vi "UIGlobalVariable.vi"(4 "Enum":enum16{"Get", "Set"}(ring), 11 "Input":T1={"Play"=FALSE, "number of samples/ch"=100000, "sound format"={"sample rate (S/s)"=22050.0, "number of channels"=2, "bits per sample"=16}}) -> (3 "Output":T1={"Play"=FALSE, "number of samples/ch"=100000, "sound format"={"sample rate (S/s)"=22050.0, "number of channels"=2, "bits per sample"=16}})   [LabVIEW 2017]
uses:
  UIData.ctl
  <vilib>/sound2/lvsound2.llb/Sound Data Format.ctl
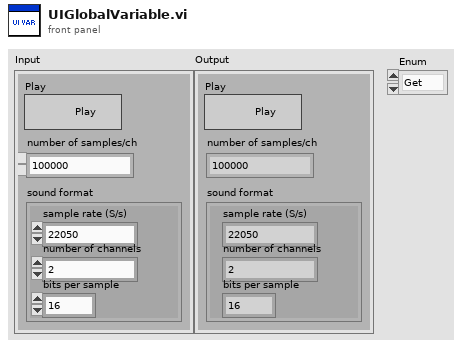
[diagram p1: front panel]
types:
  T1 = typedef "UIData.ctl" = cluster{"Play":bool, "number of samples/ch":i32, "sound format":T2}
  T2 = typedef "Sound Data Format.ctl" = cluster{"sample rate (S/s)":dbl, "number of channels":i32, "bits per sample":i32}
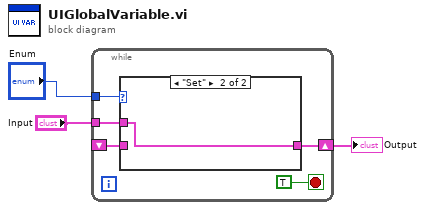
[diagram p0: block diagram]
diagram:
  n1 = while {
    tunnel: "Enum" -> [w8]
    tunnel: "Input" -> [w7]
    shift-right: [w5] -> w2
    shift-left: _ -> [w4]
    stop <- TRUE stop-if-true
    n2 = case shown="\"Set\"" w8 {
      tunnel: w7 -> [_ w10]
      tunnel: [w9 w10] -> w5
      tunnel: w4 -> [w9 _]
      frame "Get", Default {
      }
      frame "Set" {
      }
    }
  }
  "Output" <- w2
